vi "changeChannelSettings.vi"(0 "instrument handle":refnum<k15>, 1 "variant in":variant, 3 "channels":string="0", 5 "error in (no error)":errorcluster, 6 "Channel settings":T1) -> (14 "instrument handle out":refnum<k15>, 15 "Channel settings out":T1, 19 "error out":errorcluster)   [LabVIEW 2011]
uses:
  ChannelSettings_TypDef.ctl
  coupling_Enum_TypDef.ctl
  impedance_Enum_TypDEf.ctl
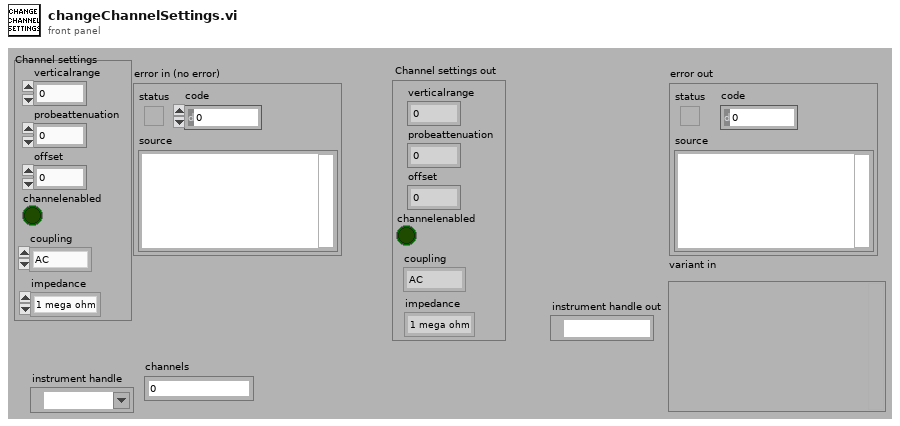
[diagram p1: front panel]
types:
  T1 = typedef "ChannelSettings_TypDef.ctl" = cluster{"verticalrange":dbl, "probeattenuation":dbl, "offset":dbl, "channelenabled":bool, "coupling":T2, "impedance":T3}
  T2 = typedef "coupling_Enum_TypDef.ctl" = enum16{"AC", "DC", "Ground"}
  T3 = typedef "impedance_Enum_TypDEf.ctl" = enum16{"1 mega ohm", "<NA>", "50 ohms"}
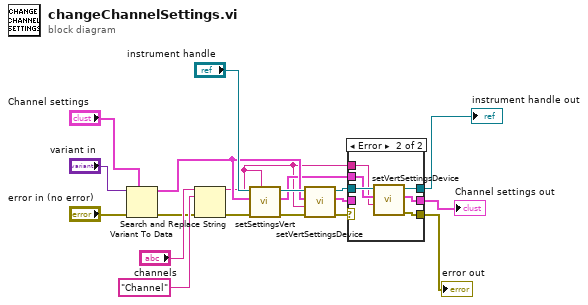
[diagram p0: block diagram]
diagram:
  n1 = Variant To Data(error in="error in (no error)", type="Channel settings", Variant="variant in") -> (data=w11:T1, error out=w14:errorcluster)
  n2 = Search and Replace String(input string="channels", search string="Channel", error in=w14) -> (result string=w5:string, error out=w2:errorcluster)  [unwired: 5 in, 2 out]
  n3 = call "setSettingsVert.vi"("Active Channel"=w5, "error out in"=w2, "Channel settings"=w11, "IVI Refnum in"="instrument handle") -> ("error out out"=w1:errorcluster, "Channel settings out"=w8:T1, "IVI Refnum out"=w12:refnum<k15>)  [unwired: 5 in]
  n4 = call "setVertSettingsDevice.vi"("error in (no error)"=w1, "Channels"=w5, "Channel settings"=w11, "IVI Refnum in"=w12) -> ("error out"=w10:errorcluster, "Channel settings out"=w6:T1, "IVI Refnum out"=w9:refnum<k15>)  [unwired: 5 in]
  n5 = case shown="Error" w10 {
    selector: w10 -> [w21 _]
    tunnel: w9 -> [w20 w28]
    tunnel: w8 -> [_ w27]
    tunnel: [w22 w26] -> w7
    tunnel: w6 -> [w22 _]
    tunnel: w5 -> [_ w25]
    tunnel: [w21 w24] -> w4
    tunnel: [w20 w23] -> w3
    frame No Error {
    }
    frame Error {
      n6 = call "setVertSettingsDevice.vi"("Channels"=w25, "Channel settings"=w27, "IVI Refnum in"=w28) -> ("error out"=w24:errorcluster, "Channel settings out"=w26:T1, "IVI Refnum out"=w23:refnum<k15>)  [unwired: 6 in]
    }
  }
  "Channel settings out" <- w7
  "error out" <- w4
  "instrument handle out" <- w3
